vi "Write Active Cell Cell Background Color.vi"(8 "error in (no error)":errorcluster, 10 "CellBGColor":u32, 11 "DigitalTable.lvclass in":refnum<class "DigitalTable.lvclass">) -> (0 "error out":errorcluster, 3 "DigitalTable.lvclass out":refnum<class "DigitalTable.lvclass">)   [LabVIEW 2015, in "DigitalTable.lvclass"]
uses:
  DigitalTable.lvclass
  DigitalTable.lvclass/DigitalTable.ctl
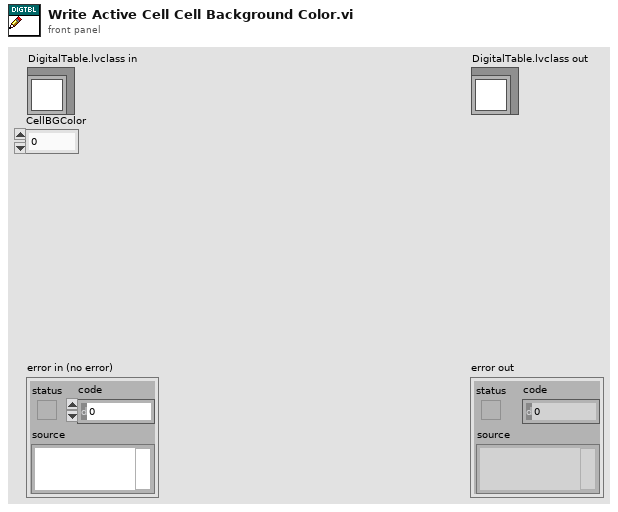
[diagram p1: front panel]
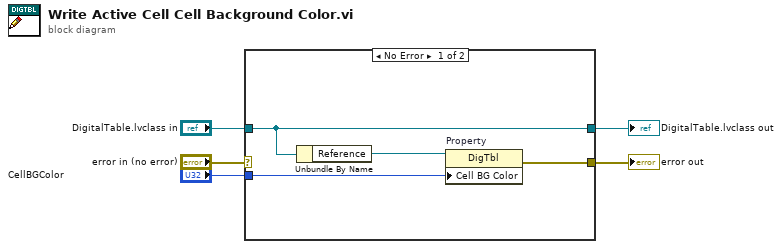
[diagram p0: block diagram]
diagram:
  n1 = case shown="No Error" "error in (no error)" {
    selector: "error in (no error)" -> [_ w11]
    tunnel: [w9 w11] -> w4
    tunnel: [w7 w10] -> w2
    tunnel: "DigitalTable.lvclass in" -> [w7 w10]
    tunnel: "CellBGColor" -> [w8 _]
    frame No Error {
      n2 = Unbundle By Name(w7) -> ("Reference"=w6:refnum<vi>)
      n3 = property on="Property" class="DigTbl"(reference=w6, "Cell BG Color"=w8) -> (error out=w9:errorcluster)  [unwired: 1 in, 1 out]
    }
    frame Error {
    }
  }
  "error out" <- w4
  "DigitalTable.lvclass out" <- w2
